vi "svx_Orbit From FString.vi"(11 "Format string":string) -> (0 "trailing zeros":bool, 1 "Precision Type":u16(ring) items=["Digits of precision", "Significant digits"], 2 "Digits":u8=1, 3 "Type":i32(listbox))   [LabVIEW 2017, in "SVX Orbit.xctl"]
uses:
  <vilib>/addons/_XControls/Orbit Plot/SVX Orbit.xctl
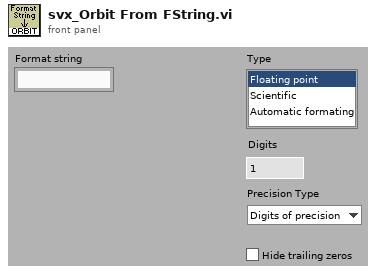
[diagram p1: front panel]
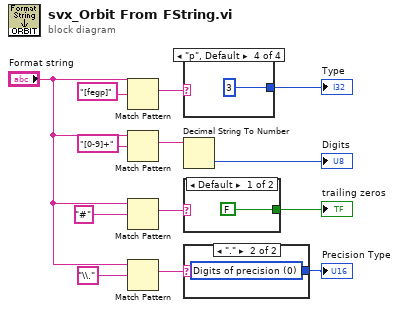
[diagram p0: block diagram]
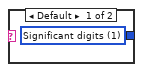
[diagram p2: hidden frame]
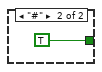
[diagram p3: hidden frame]
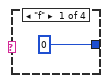
[diagram p4: hidden frame]
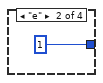
[diagram p5: hidden frame]
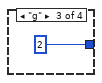
[diagram p6: hidden frame]
diagram:
  n1 = Match Pattern(string="Format string", regular expression="[fegp]" ("search string")) -> (match substring=w12:string)  [unwired: 1 in, 3 out]
  n2 = Match Pattern(string="Format string", regular expression="[0-9]+") -> (match substring=w9:string)  [unwired: 1 in, 3 out]
  n3 = Match Pattern(string="Format string", regular expression="#") -> (match substring=w6:string)  [unwired: 1 in, 3 out]
  n4 = Match Pattern(string="Format string", regular expression="\\.") -> (match substring=w2:string)  [unwired: 1 in, 3 out]
  n5 = case shown="\"p\", Default" w12 {
    tunnel: [0 ("Type") 1 ("Type") 2 ("Type") 3 ("Type")] -> w11
    frame "f" {
    }
    frame "e" {
    }
    frame "g" {
    }
    frame "p", Default {
    }
  }
  "Type" <- w11
  n6 = Decimal String To Number(string=w9) -> (number=→"Digits":i32)  [unwired: 2 in, 1 out]
  n7 = case shown="Default" w6 {
    tunnel: [FALSE ("trailing zeros") TRUE ("trailing zeros")] -> w5
    frame Default {
    }
    frame "#" {
    }
  }
  "trailing zeros" <- w5
  n8 = case shown="\".\"" w2 {
    tunnel: [w20 w21] -> w1
    frame Default {
      w20 = u16 1 items=["Digits of precision", "Significant digits"] ("Precision Type")
    }
    frame "." {
      w21 = u16 0 items=["Digits of precision", "Significant digits"] ("Precision Type")
    }
  }
  "Precision Type" <- w1
